vi "ACT_FlowDiagrams2.vi"() -> ()   [LabVIEW 2016]
panel:
  out "Result":dbl
  in  "Numeric":dbl
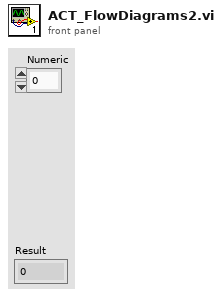
[diagram p1: front panel]
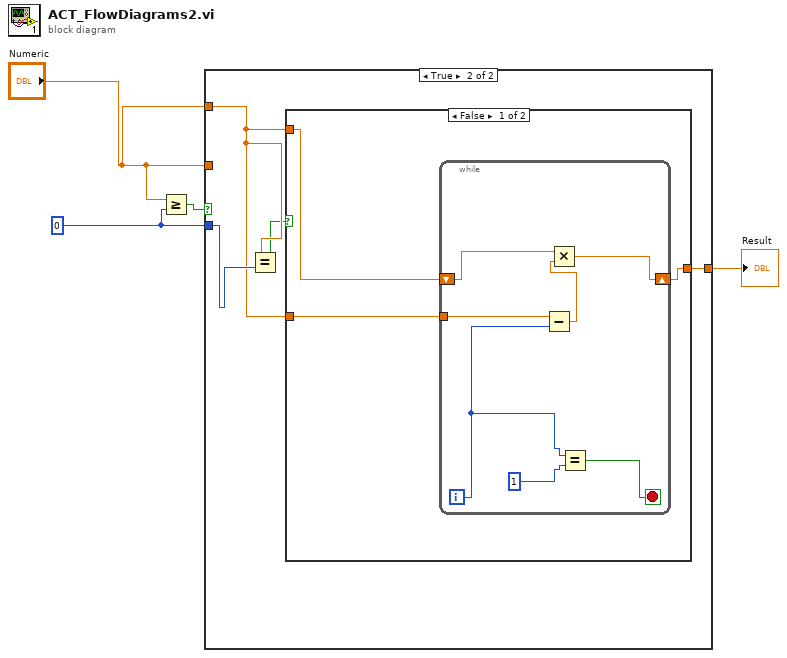
[diagram p0: block diagram]
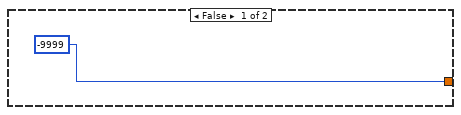
[diagram p2: hidden frame]
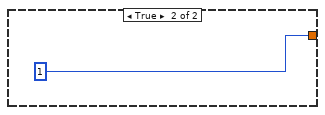
[diagram p3: hidden frame]
diagram:
  w2 = 0
  n1 = Greater Or Equal?(x="Numeric", y=w2) -> (x >= y?=w1:bool)
  n2 = case shown="True" w1 {
    tunnel: "Numeric" -> [_ w7]
    tunnel: [-9999 w9] -> w4
    tunnel: "Numeric" -> [_ _]
    tunnel: w2 -> [_ w8]
    frame False {
    }
    frame True {
      n3 = Equal?(x=w7, y=w8) -> (x = y?=w6:bool)
      n4 = case shown="False" w6 {
        tunnel: w7 -> [w12 _]
        tunnel: [w11 1] -> w9
        tunnel: w7 -> [w10 _]
        frame False {
          n5 = while {
            shift-right: [w17] -> w11
            shift-left: w10 -> [w19]
            tunnel: w12 -> [w16]
            i -> [w15]
            stop <- w13 stop-if-true
            n6 = Subtract(x=w16, y=w15) -> (x-y=w18:dbl)
            n7 = Multiply(x=w19, y=w18) -> (x*y=w17:dbl)
            n8 = Equal?(x=w15, y=1) -> (x = y?=w13:bool)
          }
        }
        frame True {
        }
      }
    }
  }
  "Result" <- w4
